vi "SMO.LaunchDependency.vi"(6 "Shared Resource":bool, 7 "Level":string, 8 "error in (no error)":errorcluster, 9 "Dependency Name":string, 10 "Dependency Type":refnum<class "SMO.lvclass">, 11 "SMO in":refnum<class "SMO.lvclass">) -> (0 "error out":errorcluster, 1 "Unique Name":string, 3 "SMO out":refnum<class "SMO.lvclass">)   [LabVIEW 2013, in "SMO.lvclass"]
uses:
  SMO.lvclass
  Support/Attribute.Owner/Attribute.Owner.lvclass/Attribute.Owner.ctl
  Support/Attribute.SharedResource/Attribute.SharedResource.lvclass
  Support/Attribute.Owner/Attribute.Owner.lvclass
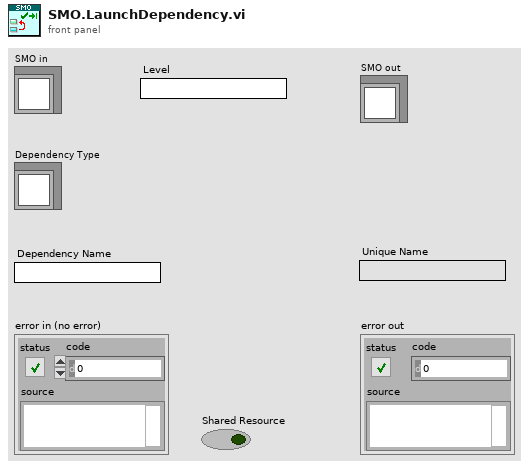
[diagram p1: front panel]
types:
  T1 = typedef "SMO.lvclass/SMOState --Enum.ctl" = enum16{"unknown", "Created", "Started", "Stopped"}
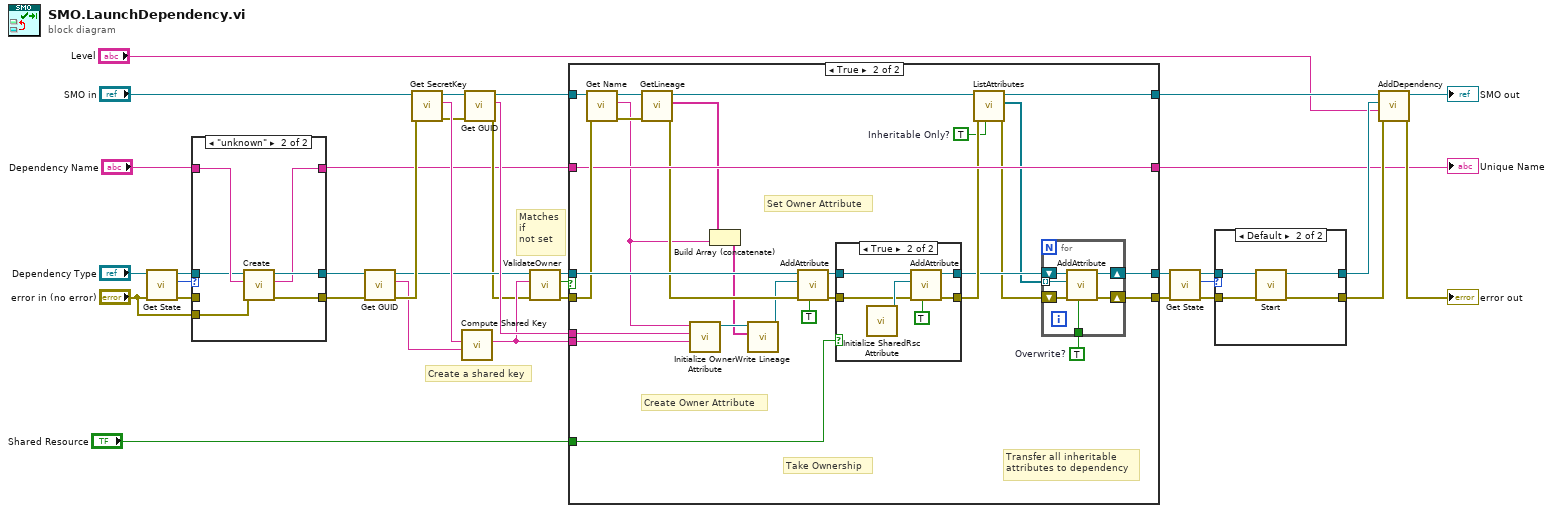
[diagram p0: block diagram]
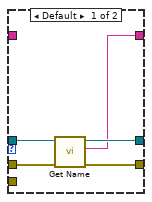
[diagram p5: hidden frame]
diagram:
  # "Matches\nif\nnot set"
  # "Create a shared key"
  n1 = call "Get State.vi"("error in (no error)"="error in (no error)", "SMO"="Dependency Type") -> ("error out"=w21:errorcluster, "SMO State"=w20:T1, "SMO out"=w22:refnum<class "SMO.lvclass">)  [unwired: 7 in]
  n2 = case shown="\"unknown\"" w20 {
    tunnel: [w38 w47] -> w26
    tunnel: [w39 w46] -> w25
    tunnel: "Dependency Name" -> [_ w45]
    tunnel: [w37 w44] -> w4
    tunnel: w22 -> [w41 w43]
    tunnel: w21 -> [w40 _]
    tunnel: "error in (no error)" -> [_ w42]
    frame Default {
      n3 = call "Get Name.vi"("error in (no error)"=w40, "SMO"=w41) -> ("error out"=w38:errorcluster, "Name"=w37:string, "SMO out"=w39:refnum<class "SMO.lvclass">)  [unwired: 7 in]
    }
    frame "unknown" {
      n4 = call "Create.vi"("error in (no error)"=w42, "Subsystem Name (optional)"=w45, "SMO"=w43) -> ("error out"=w47:errorcluster, "SMO name"=w44:string, "SMO out"=w46:refnum<class "SMO.lvclass">)  [unwired: 6 in]
    }
  }
  n5 = call "Get GUID.vi"("error in (no error)"=w26, "SMO"=w25) -> ("error out"=w34:errorcluster, "GUID"=w27:string, "SMO out"=w10:refnum<class "SMO.lvclass">)  [unwired: 7 in]
  n6 = call "Get SecretKey.vi"("error in (no error)"=w34, "SMO"="SMO in") -> ("error out"=w30:errorcluster, "SecretKey"=w36:string, "SMO out"=w31:refnum<class "SMO.lvclass">)  [unwired: 7 in]
  n7 = call "Compute Shared Key.vi"("GUID"=w27, "SecretKey"=w36) -> ("Shared Key"=w8:string)  [unwired: 9 in]
  n8 = call "Get GUID.vi"("error in (no error)"=w30, "SMO"=w31) -> ("error out"=w7:errorcluster, "GUID"=w35:string, "SMO out"=w32:refnum<class "SMO.lvclass">)  [unwired: 7 in]
  n9 = call "ValidateOwner.vi"("error in (no error)"=w7, "Shared Key"=w8, "SMO in"=w10) -> ("error out"=w6:errorcluster, "key matched"=w5:bool, "SMO out"=w9:refnum<class "SMO.lvclass">)  [unwired: 6 in]
  n10 = case shown="True" w5 {
    tunnel: w35 -> [_ w79]
    tunnel: [w51 w70] -> w33
    tunnel: w32 -> [w51 w78]
    tunnel: "Shared Resource" -> [_ w77]
    tunnel: [w50 w67] -> w14
    tunnel: [w49 w64] -> w12
    tunnel: w9 -> [w50 w74]
    tunnel: w8 -> [_ w73]
    tunnel: w6 -> [w49 w72]
    tunnel: w4 -> [w48 w71]
    tunnel: [w48 w71] -> w3
    frame False {
      # "Already Owned by other SMO"
    }
    frame True {
      w63 = TRUE  # Overwrite?
      w68 = TRUE  # Inheritable Only?
      # "Transfer all inheritable\nattributes to dependency"
      # "Take Ownership"
      # "Create Owner Attribute"
      # "Set Owner Attribute"
      n11 = call "Get Name.vi"("error in (no error)"=w72, "SMO"=w78) -> ("error out"=w58:errorcluster, "Name"=w53:string, "SMO out"=w60:refnum<class "SMO.lvclass">)  [unwired: 7 in]
      n12 = call "GetLineage.vi"("error in (no error)"=w58, "SMO in"=w60) -> ("error out"=w57:errorcluster, "Lineage"=w54:string[], "SMO out"=w59:refnum<class "SMO.lvclass">)  [unwired: 7 in]
      n13 = call "Initialize Owner Attribute.vi"("Shared Key"=w73, "Owner GUID"=w79, "Owner Name"=w53) -> ("Attribute.Owner"=w56:refnum<class "Attribute.Owner.lvclass">)  [unwired: 8 in]
      n14 = Build Array (concatenate)(w54, w53) -> (w52:string[])
      n15 = call "Write Lineage.vi"("Lineage"=w52, "Attribute.Owner in"=w56) -> ("Attribute.Owner out"=w55:refnum<class "Attribute.Owner.lvclass">)  [unwired: 8 in, 1 out]
      n16 = call "AddAttribute.vi"("Overwrite? (F)"=TRUE, "error in (no error)"=w57, "Attribute"=w55, "SMO in"=w74) -> ("error out"=w76:errorcluster, "SMO out"=w75:refnum<class "SMO.lvclass">)  [unwired: 6 in]
      n17 = case shown="True" w77 {
        tunnel: w75 -> [w87 w93]
        tunnel: [w87 w92] -> w66
        tunnel: w76 -> [w86 w90]
        tunnel: [w86 w89] -> w69
        frame False {
        }
        frame True {
          n18 = call "Initialize SharedRsc Attribute.vi"() -> ("Attribute.SharedResource"=w91:refnum<class "Attribute.SharedResource.lvclass">)  [unwired: 11 in]
          n19 = call "AddAttribute.vi"("Overwrite? (F)"=TRUE, "error in (no error)"=w90, "Attribute"=w91, "SMO in"=w93) -> ("error out"=w89:errorcluster, "SMO out"=w92:refnum<class "SMO.lvclass">)  [unwired: 6 in]
        }
      }
      n20 = call "ListAttributes.vi"("Inheritable Only? (F: all)"=w68, "error in (no error)"=w69, "SMO in"=w59) -> ("error out"=w65:errorcluster, "[Attributes]"=w62:refnum<class "Attribute.lvclass">[], "SMO out"=w70:refnum<class "SMO.lvclass">)  [unwired: 6 in]
      n21 = for {
        tunnel: w63 -> [w81]
        shift-right: [w85] -> w67
        shift-left: w66 -> [w84]
        shift-right: [w82] -> w64
        shift-left: w65 -> [w83]
        tunnel: w62 -> [w80] mode=indexing
        n22 = call "AddAttribute.vi"("Overwrite? (F)"=w81, "error in (no error)"=w83, "Attribute"=w80, "SMO in"=w84) -> ("error out"=w82:errorcluster, "SMO out"=w85:refnum<class "SMO.lvclass">)  [unwired: 6 in]
      }
    }
  }
  "Unique Name" <- w3
  n23 = call "Get State.vi"("error in (no error)"=w12, "SMO"=w14) -> ("error out"=w13:errorcluster, "SMO State"=w11:T1, "SMO out"=w15:refnum<class "SMO.lvclass">)  [unwired: 7 in]
  n24 = case shown="Default" w11 {
    tunnel: [w94 w99] -> w17
    tunnel: [w95 w98] -> w16
    tunnel: w15 -> [w95 w97]
    tunnel: w13 -> [w94 w96]
    frame "Started" {
    }
    frame Default {
      n25 = call "Start.vi"("error in (no error)"=w96, "SMO"=w97) -> ("error out"=w99:errorcluster, "SMO out"=w98:refnum<class "SMO.lvclass">)  [unwired: 8 in]
    }
  }
  n26 = call "AddDependency.vi"("error in (no error)"=w17, "Level"="Level", "Dependency"=w16, "SMO in"=w33) -> ("error out"=→"error out":errorcluster, "SMO out"=→"SMO out":refnum<class "SMO.lvclass">)  [unwired: 6 in]
